vi "Write Vss Tactics.vi"(8 "error in (no error)":errorcluster, 10 "Vss Tactics":T1, 11 "Tacticbook in":refnum<class "Tacticbook.lvclass">) -> (0 "error out":errorcluster, 3 "Tacticbook out":refnum<class "Tacticbook.lvclass">)   [LabVIEW 2018, in "Tacticbook.lvclass"]
uses:
  Tacticbook.lvclass
  DispBallTacticVSS_class/DispBallTacticVSS.lvclass
  DefendGoalTacticVSS_class/DefendGoalTacticVSS.lvclass
  PenaltyAttackTacticVSS_class/PenaltyAttackTacticVSS.lvclass
  DefendAreaTacticVSS_class/DefendAreaTacticVSS.lvclass
  AttackTacticVSS_class/AttackTacticVSS.lvclass
  HaltTactic_class/HaltTactic.lvclass
  Tacticbook.lvclass/Tacticbook.ctl
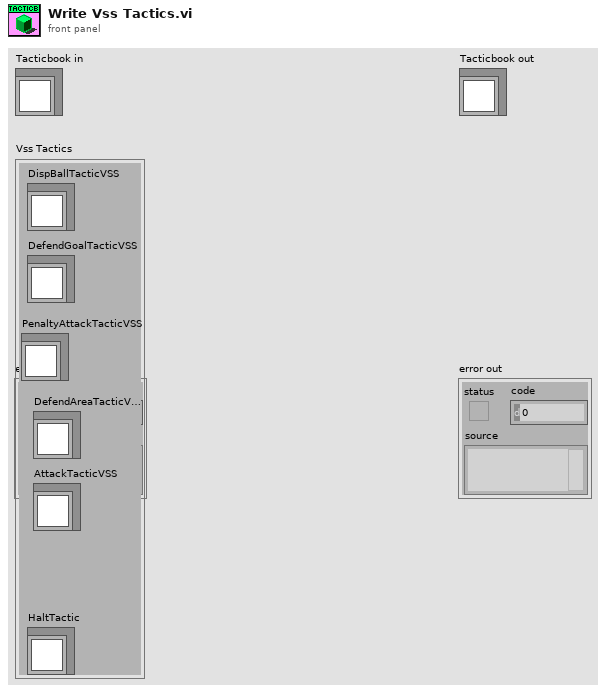
[diagram p1: front panel]
types:
  T1 = cluster{"DispBallTacticVSS":refnum<class "DispBallTacticVSS.lvclass">, "DefendGoalTacticVSS":refnum<class "DefendGoalTacticVSS.lvclass">, "PenaltyAttackTacticVSS":refnum<class "PenaltyAttackTacticVSS.lvclass">, "DefendAreaTacticVSS":refnum<class "DefendAreaTacticVSS.lvclass">, "AttackTacticVSS":refnum<class "AttackTacticVSS.lvclass">, "HaltTactic":refnum<class "HaltTactic.lvclass">}
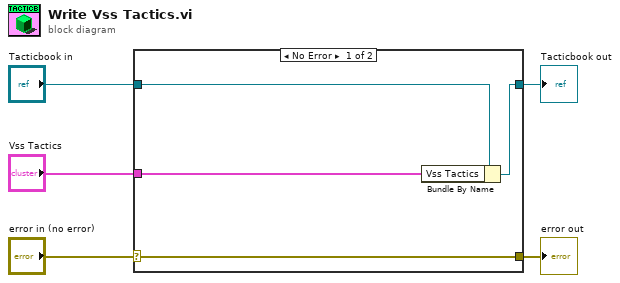
[diagram p0: block diagram]
diagram:
  n1 = case shown="No Error" "error in (no error)" {
    selector: "error in (no error)" -> [w9 w10]
    tunnel: [w9 w10] -> w4
    tunnel: [w7 w11] -> w2
    tunnel: "Tacticbook in" -> [w8 w11]
    tunnel: "Vss Tactics" -> [w6 _]
    frame No Error {
      n2 = Bundle By Name(cluster=w8, "Vss Tactics"=w6) -> (w7:refnum<class "Tacticbook.lvclass">)
    }
    frame Error {
    }
  }
  "error out" <- w4
  "Tacticbook out" <- w2
